vi "GetPos.vi"(6 "Position 2":refnum<vi>, 8 "error in (no error)":errorcluster, 11 "Motor in":refnum<class "Motor.lvclass">) -> (0 "error out":errorcluster, 2 "Position":dbl, 3 "Motor out":refnum<class "Motor.lvclass">)   [LabVIEW 2012, in "Motor.lvclass"]
uses:
  Motor.lvclass
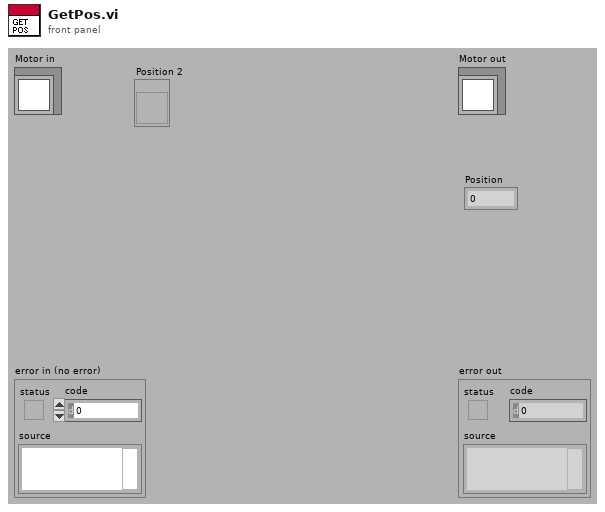
[diagram p1: front panel]
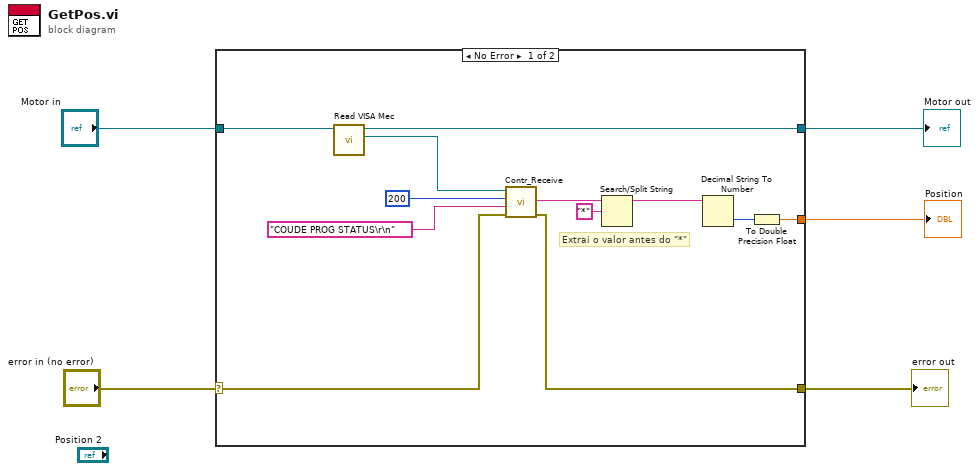
[diagram p0: block diagram]
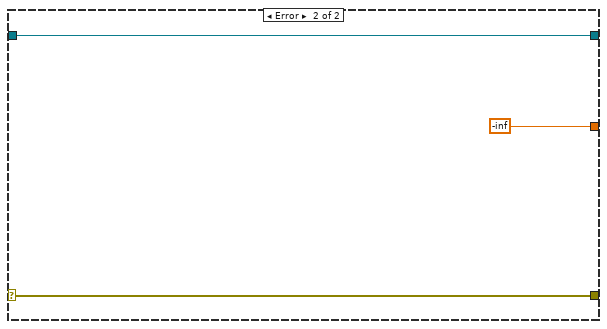
[diagram p2: hidden frame]
diagram:
  n1 = case shown="No Error" "error in (no error)" {
    selector: "error in (no error)" -> [w12 w19]
    tunnel: "Motor in" -> [w16 w20]
    tunnel: [w15 w20] -> w2
    tunnel: [w11 w19] -> w3
    tunnel: [w6 -inf] -> w1
    frame No Error {
      # "Extrai o valor antes do \"*\""
      n2 = call-dynamic "Read VISA Mec.vi"("Controlador in"=w16) -> ("VISA Mec"=w14:refnum<visa-resource-name>, "Controlador out"=w15:refnum<class "Motor.lvclass">)  [unwired: 8 in, 1 out]
      n3 = call "Contr_Receive.vi"("error in"=w12, "Command to SIFS"="COUDE PROG STATUS\r\n", "wait after tx"=u32 200, "VISA resource name"=w14) -> ("error out"=w11:errorcluster, "Response from SIFS"=w10:string)  [unwired: 2 out]
      n4 = Search/Split String(string=w10, search string/char (-)="*") -> (substring before match=w8:string)  [unwired: 1 in, 2 out]
      n5 = Decimal String To Number(string=w8) -> (number=w7:i32)  [unwired: 2 in, 1 out]
      n6 = To Double Precision Float(number=w7) -> (double precision float=w6:dbl)
    }
    frame Error {
    }
  }
  "error out" <- w3
  "Motor out" <- w2
  "Position" <- w1
